vi "MeansOfData.vi"(10 "var":sgl[][][](array[numeric]), 11 "pow":sgl[][][](array[numeric])) -> (1 "mean var":sgl[][](array[numeric]), 2 "mean pow":sgl[][](array[numeric]), 3 "rms":dbl[][](array[numeric]))   [LabVIEW 2022 SP3]
uses:
  <vilib>/Analysis/baseanly.llb/Mean (DBL).vi
  <vilib>/Analysis/NI_AALBase.lvlib
  <vilib>/Analysis/NI_AALPro.lvlib
panel:
  out "Median Pow":dbl[][](graph)
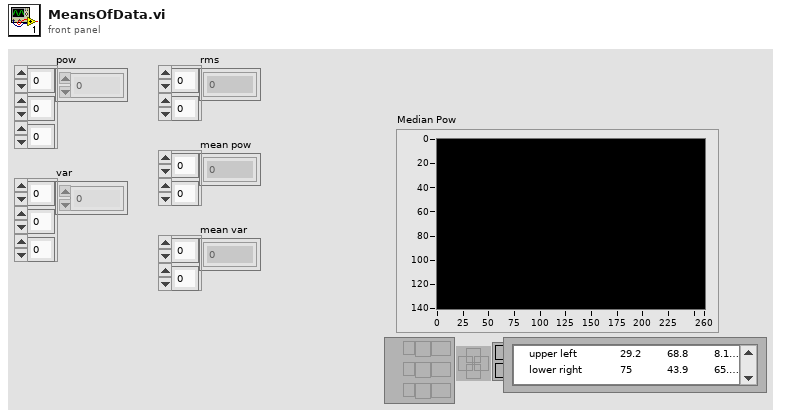
[diagram p1: front panel]
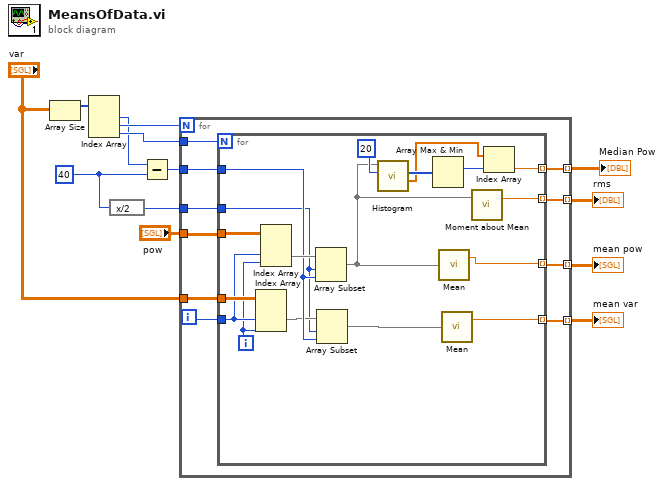
[diagram p0: block diagram]
diagram:
  w5 = 40 ("y")
  n1 = Array Size(array="var") -> (size(s)=w8:i32[])
  n2 = Index Array(array=w8) -> (element #1=w6:i32, element #2=w11:i32, element #3=w10:i32)  [unwired: 3 in]
  n3 = expression code="x/2"(w5) -> (w4:i32)
  n4 = Subtract(x=w6, y=w5) -> (x-y=w3:i32)
  n5 = for {
    N: w11 -> [_]
    tunnel: "var" -> [w22]
    tunnel: w10 -> [w23]
    tunnel: [w20] -> w9 mode=indexing
    tunnel: "pow" -> [w19]
    tunnel: [w18] -> w13 mode=indexing
    tunnel: [w17] -> w2 mode=indexing
    tunnel: w4 -> [w16]
    tunnel: w3 -> [w15]
    tunnel: [w14] -> w1 mode=indexing
    i -> [w21]
    n6 = for {
      N: w23 -> [_]
      tunnel: w22 -> [w41]
      tunnel: w21 -> [w39]
      tunnel: [w36] -> w20 mode=indexing
      tunnel: w19 -> [w40]
      tunnel: [w37] -> w18 mode=indexing
      tunnel: [w31] -> w17 mode=indexing
      tunnel: w16 -> [w32]
      tunnel: w15 -> [w34]
      tunnel: [w25] -> w14 mode=indexing
      i -> [w38]
      n7 = Index Array(array=w41, index (dim 1)=w39, index (dim 2)=w38) -> (element=w33:sgl[])  [unwired: 1 in]
      n8 = Index Array(array=w40, index (dim 1)=w39, index (dim 2)=w38) -> (element=w35:sgl[])  [unwired: 1 in]
      n9 = Array Subset(array=w35, index=w32, length=w34) -> (w24:sgl[])
      n10 = Array Subset(array=w33, index=w32, length=w34) -> (w29:sgl[])
      n11 = call <vilib>:"Histogram.vi"("intervals"=20, "X"=w24) -> ("X Values"=w26:dbl[], "Histogram: h(x)"=w28:i32[])  [unwired: 6 in, 2 out]
      n12 = Array Max & Min(array=w28) -> (max index (indices)=w27:i32)  [unwired: 3 out]
      n13 = call-poly <vilib>:"Mean.vi"("X"=w24) -> ("mean"=w37:dbl)  [unwired: 1 out]
      n14 = call-poly <vilib>:"Mean.vi"("X"=w29) -> ("mean"=w36:dbl)  [unwired: 1 out]
      n15 = call <vilib>:"Moment about Mean.vi"("X"=w24) -> ("moment"=w31:dbl)  [unwired: 1 in, 1 out]
      n16 = Index Array(array=w26, index=w27) -> (element=w25:dbl)
    }
  }
  "rms" <- w2
  "mean pow" <- w13
  "mean var" <- w9
  "Median Pow" <- w1
